vi "Send Configure Glitch Trigger Source [GT].vi"(4 "glitch condition (Less Than)":i32(ring)=1 items=["Less Than"=1, "Greater Than"=2], 5 "glitch polarity (Positive)":i32(ring)=1 items=["Positive"=1, "Negative"=2, "Either"=3], 6 "glitch width (10 ms)":dbl[unit]=1e-05 format="%^.2e", 7 "Message Priority (Normal)":T1=enum."Normal", 8 "error in (no error)":errorcluster, 9 "trigger level (0.0 V)":dbl[unit] format="%.3f", 10 "trigger source (\"CHANNEL1\")":string(combo)="CHANNEL1", 11 "Message Enqueuer":refnum<class "Message Enqueuer.lvclass">) -> (0 "error out":errorcluster, 3 "Message Enqueuer out":refnum<class "Message Enqueuer.lvclass">)   [LabVIEW 2016, in "CS++Scope.lvlib" / "Configure Glitch Trigger Source [GT] Msg.lvclass"]
doc: "Sends the <B>CS++Scope.lvlib:Configure Glitch Trigger Source [GT] Msg.lvclass</B> message.\n\n<B>CS++Scope.lvlib:CS++Scope.lvclass:Configure Glitch Trigger Source [GT].vi</B> Description:\n\nThis VI configures the glitch trigger. A glitch trigger occurs when the trigger signal has a pulse with a width that is less than or greater than the glitch width. You specifiy which comparison criterion to use with the glitchCondition parameter. You specifiy the glitch width in the glitchWidth parameter. You specifiy the polarity of the pulse with the glitchPolarity parameter. The trigger does not actually occur until the edge of a pulse that corresponds to the glitchWidth and glitchPolarity crosses the threshold the end-user specifies in the triggerLevel parameter.\n\nNote:\nThis VI affects instrument behavior only if the trigger type is IVISCOPE_VAL_GLITCH_TRIGGER. Call the IviScope Configure Trigger and IviScope Configure Trigger Coupling VIs to set the trigger type and trigger coupling before calling this VI."
uses:
  Configure Glitch Trigger Source [GT] Msg.lvclass
  <vilib>/ActorFramework/Message Enqueuer/Message Enqueuer.lvclass
  <vilib>/ActorFramework/Message Enqueuer/Message Priority.ctl
  C:/Program Files (x86)/National Instruments/LabVIEW 2016/vi.lib/ActorFramework/Message/Message.lvclass
  Configure Glitch Trigger Source [GT] Msg.lvclass/Configure Glitch Trigger Source [GT] Msg.ctl
  <vilib>/ActorFramework/Message Enqueuer/Message Enqueuer.lvclass/Message Enqueuer.ctl
  <vilib>/ActorFramework/Message Priority Queue/Priority Enqueue.vi
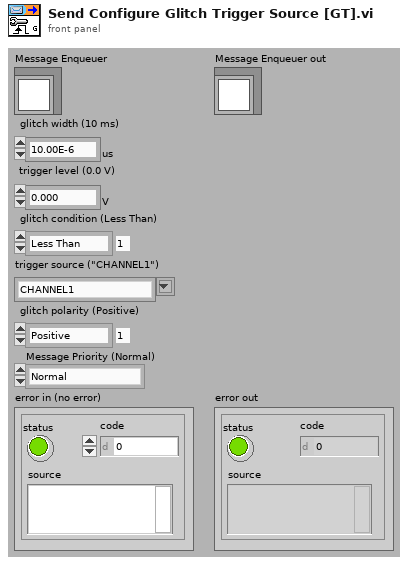
[diagram p1: front panel]
types:
  T1 = typedef "Actor Framework.lvlib/Message Enqueuer.lvclass/Message Priority.ctl" = enum16{"Low", "Normal", "High"}
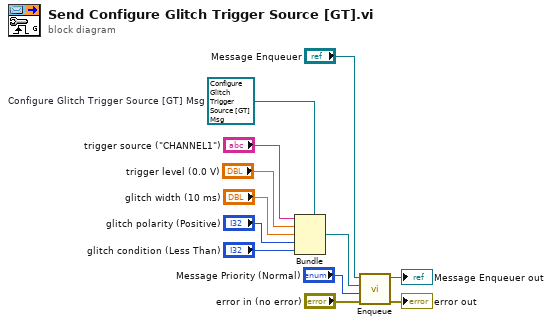
[diagram p0: block diagram]
diagram:
  w6 = refnum<class "Configure Glitch Trigger Source [GT] Msg.lvclass"> refnum  # Configure Glitch Trigger Source [GT] Msg
  n1 = Bundle(cluster=w6, "trigger source (\"CHANNEL1\")", "trigger level (0.0 V)", "glitch width (10 ms)", "glitch polarity (Positive)", "glitch condition (Less Than)") -> (w9:refnum<class "Configure Glitch Trigger Source [GT] Msg.lvclass">)
  n2 = call <vilib>:"Enqueue.vi"("error in (no error)"="error in (no error)", "Message Priority (Normal)"="Message Priority (Normal)", "Message"=w9, "Message Enqueuer in"="Message Enqueuer") -> ("error out"=→"error out":errorcluster, "Message Enqueuer out"=→"Message Enqueuer out":refnum<class "Message Enqueuer.lvclass">)  [unwired: 6 in]
